vi "Close.vi"(8 "error in":errorcluster, 11 "Power Gradient in":refnum<class "Power Gradient.lvclass">) -> (0 "error out":errorcluster, 3 "Power Gradient out":refnum<class "Power Gradient.lvclass">)   [LabVIEW 2023, in "Power Gradient.lvclass"]
uses:
  Power Gradient.lvclass
  Power Gradient.lvclass/Power Gradient.ctl
  Parents/Gradient/Gradient.lvclass
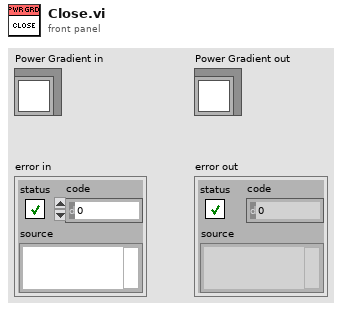
[diagram p1: front panel]
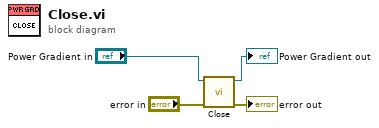
[diagram p0: block diagram]
diagram:
  n1 = call-parent "Close.vi"("error in"="error in", "Gradient in"="Power Gradient in") -> ("error out"=→"error out":errorcluster, "Gradient out"=→"Power Gradient out":refnum<class "Power Gradient.lvclass">)  [unwired: 8 in]
